vi "InterpretPacket.vi"(11 "Data In":string) -> (3 "Data Out":u8, 5 "output cluster":T1)   [LabVIEW 2009]
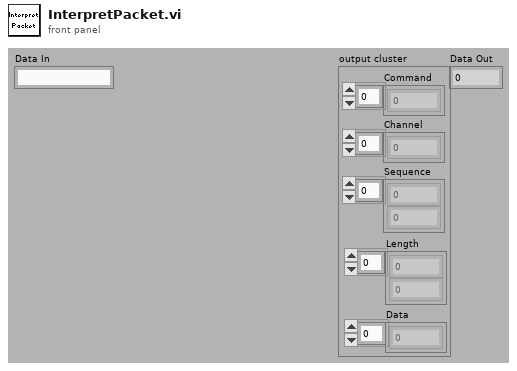
[diagram p1: front panel]
types:
  T1 = cluster{"Command":i32[], "Channel":i32[], "Sequence":i32[], "Length":i32[], "Data":i32[]}
  T2 = cluster{"Command":u8[], "Channel":u8[], "Sequence":u8[], "Length":u8[], "Data":u8[]}
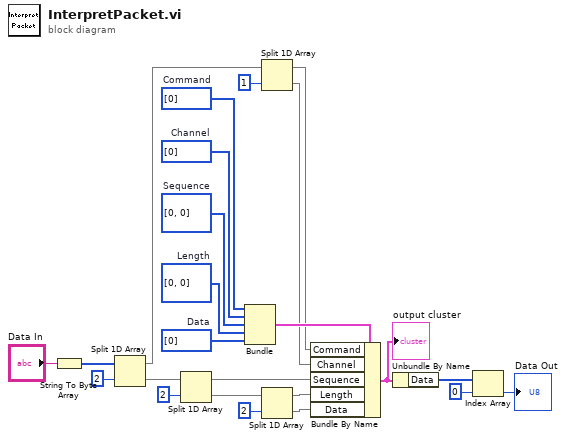
[diagram p0: block diagram]
diagram:
  w14 = u8[] [0]  # Channel
  w13 = u8[] [0, 0]  # Sequence
  w12 = u8[] [0, 0]  # Length
  w11 = u8[] [0]  # Data
  w15 = u8[] [0]  # Command
  n1 = String To Byte Array(string="Data In") -> (unsigned byte array=w23:u8[])
  n2 = Split 1D Array(array=w23, index=2) -> (first subarray=w19:u8[], second subarray=w21:u8[])
  n3 = Split 1D Array(array=w21, index=2) -> (first subarray=w7:u8[], second subarray=w17:u8[])
  n4 = Bundle("Command"=w15, "Channel"=w14, "Sequence"=w13, "Length"=w12, "Data"=w11) -> (w10:T2)  [unwired: 1 in]
  n5 = Split 1D Array(array=w19, index=1) -> (first subarray=w9:u8[], second subarray=w8:u8[])
  n6 = Split 1D Array(array=w17, index=2) -> (first subarray=w6:u8[], second subarray=w5:u8[])
  n7 = Bundle By Name(cluster=w10, "Command"=w9, "Channel"=w8, "Sequence"=w7, "Length"=w6, "Data"=w5) -> (w4:T2)
  "output cluster" <- w4
  n8 = Unbundle By Name(w4) -> ("Data"=w3:u8[])
  n9 = Index Array(array=w3, index=0) -> (element=→"Data Out":u8)
